vi "dump.vi"(8 "error in (no error)":errorcluster, 10 "indent":T1, 11 "StringLiteral in":refnum<class "StringLiteral.lvclass">) -> (0 "error out":errorcluster, 2 "mlir":string, 3 "StringLiteral out":refnum<class "StringLiteral.lvclass">)   [LabVIEW 2020, in "mlir.lvlib" / "StringLiteral.lvclass"]
uses:
  StringLiteral.lvclass
  Node/indent.ctl
  StringLiteral.lvclass/StringLiteral.ctl
  mlir.lvlib
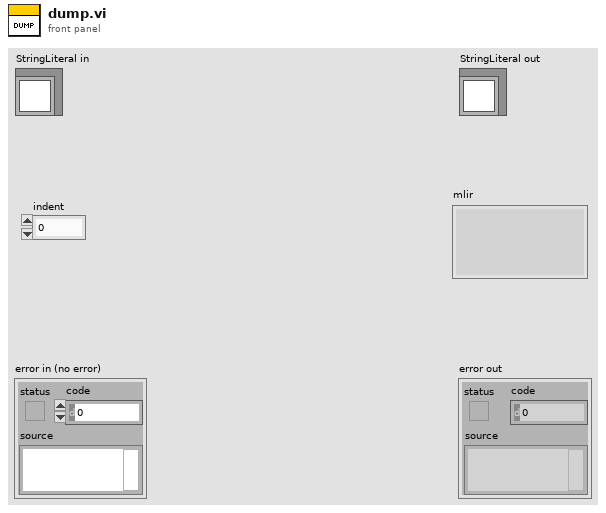
[diagram p1: front panel]
types:
  T1 = typedef "mlir.lvlib/indent.ctl" = u32
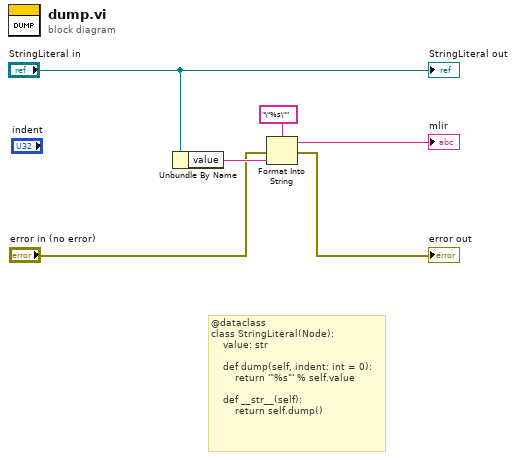
[diagram p0: block diagram]
diagram:
  # "@dataclass\nclass StringLiteral(Node):\n    value: str\n\n    def dump(self, indent: int = 0):\n        return '\"%s\"' % self.value\n\n    def __str__(self):\n        return self.dump()"
  n1 = Unbundle By Name("StringLiteral in") -> ("value"=w5:string)
  n2 = Format Into String(format string="\"%s\"", error in="error in (no error)", w5) -> (resulting string=→"mlir":string, error out=→"error out":errorcluster)  [unwired: 1 in]
  "StringLiteral out" <- "StringLiteral in"
